vi "Get Child Attributes.vi"(0 "Linked List in":refnum<class "Linked List.lvclass">, 1 "Linked List ID":string, 5 "IDs":string[](array[string]), 7 "Missing GUIDs":string[](array[string]), 9 "Attributes":variant[](array[variant]), 11 "error in (no error)":errorcluster, 12 "Names":string[](array[string])) -> (3 "Linked List ID out":string, 4 "Linked List out":refnum<class "Linked List.lvclass">, 6 "IDs":string[](array[string]), 8 "Missing GUIDs out":string[](array[string]), 10 "Attributes":variant[](array[variant]), 14 "Names":string[](array[string]), 15 "error out":errorcluster)   [LabVIEW 2020, in "Linked Lists.lvlib" / "Linked List.lvclass"]
uses:
  <vilib>/gpm_packages/@cs/linked-list/Source/Linked List/Linked List/Linked List.lvclass
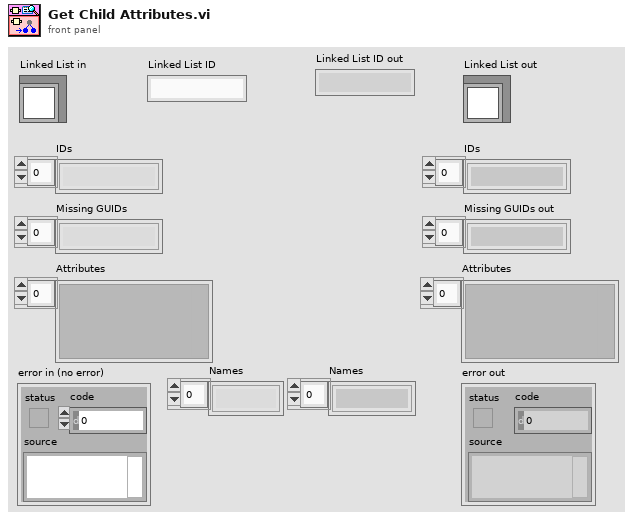
[diagram p1: front panel]
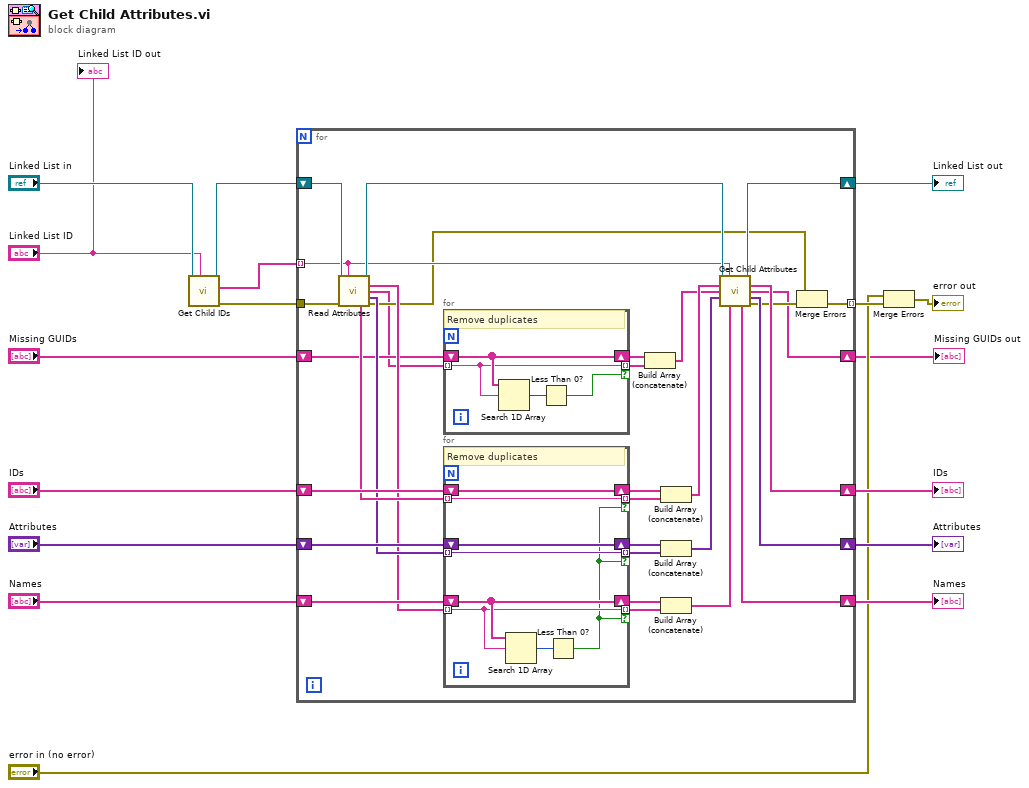
[diagram p0: block diagram]
diagram:
  n1 = call-dynamic "Get Child IDs.vi"("Linked List ID"="Linked List ID", "Linked List in"="Linked List in") -> ("error out"=w5:errorcluster, "Child IDs"=w6:string[], "Linked List out"=w7:refnum<class "Linked List.lvclass">)  [unwired: 7 in]
  n2 = for {
    shift-right: [w46] -> w15
    shift-left: w7 -> [w48]
    tunnel: w6 -> [w45] mode=indexing
    shift-right: [w43] -> w8
    shift-left: "Names" -> [w29]
    shift-right: [w41] -> w9
    shift-left: "Attributes" -> [w33]
    shift-right: [w39] -> w10
    shift-left: "IDs" -> [w37]
    tunnel: w5 -> [w49]
    tunnel: [w25] -> w17 mode=indexing
    shift-right: [w18] -> w1
    shift-left: "Missing GUIDs" -> [w23]
    n3 = call-dynamic "Read Attributes.vi"("Linked List in"=w48, "Linked List ID"=w45, "error in (no error)"=w49) -> ("Linked List out"=w47:refnum<class "Linked List.lvclass">, "Attribute Names out"=w27:string[], "Missing GUIDs out"=w22:string[], "Attributes"=w31:variant[], "Data IDs"=w35:string[], "error out"=w24:errorcluster)  [unwired: 6 in, 1 out]
    n4 = for {
      shift-right: [w52] -> w21
      shift-left: w23 -> [w52]
      tunnel: w22 -> [w51] mode=indexing
      tunnel: [w51] -> w20 mode=indexing if=w50
      # "Remove duplicates"
      n5 = Search 1D Array(1D array=w52, element=w51) -> (index of element=w53:i32)  [unwired: 1 in]
      n6 = Less Than 0?(x=w53) -> (x < 0?=w50:bool)
    }
    n7 = for {
      shift-right: [w61] -> w36
      shift-left: w37 -> [w61]
      tunnel: [w60] -> w34 mode=indexing if=w54
      tunnel: w35 -> [w60] mode=indexing
      shift-right: [w59] -> w32
      shift-left: w33 -> [w59]
      tunnel: w31 -> [w58] mode=indexing
      tunnel: [w58] -> w30 mode=indexing if=w54
      shift-right: [w57] -> w28
      shift-left: w29 -> [w57]
      tunnel: w27 -> [w56] mode=indexing
      tunnel: [w56] -> w26 mode=indexing if=w54
      # "Remove duplicates"
      n8 = Search 1D Array(1D array=w57, element=w56) -> (index of element=w55:i32)  [unwired: 1 in]
      n9 = Less Than 0?(x=w55) -> (x < 0?=w54:bool)
    }
    n10 = Build Array (concatenate)(w21, w20) -> (w19:string[])
    n11 = Build Array (concatenate)(w36, w34) -> (w40:string[])
    n12 = Build Array (concatenate)(w32, w30) -> (w42:variant[])
    n13 = Build Array (concatenate)(w28, w26) -> (w44:string[])
    n14 = call <vilib>:"Get Child Attributes.vi"("Linked List in"=w47, "Linked List ID"=w45, "IDs"=w40, "Missing GUIDs"=w19, "Attributes"=w42, "Names"=w44) -> ("Linked List out"=w46:refnum<class "Linked List.lvclass">, "IDs"=w39:string[], "Missing GUIDs out"=w18:string[], "Attributes"=w41:variant[], "Names"=w43:string[], "error out"=w38:errorcluster)  [unwired: 3 in, 1 out]
    n15 = Merge Errors(w24, w38) -> (w25:errorcluster)
  }
  "Linked List out" <- w15
  "IDs" <- w10
  "Attributes" <- w9
  "Names" <- w8
  "Missing GUIDs out" <- w1
  n16 = Merge Errors("error in (no error)", w17) -> (→"error out":errorcluster)
  "Linked List ID out" <- "Linked List ID"
